vi "displayConfigurableElements.vi"(11 "ConfigurationThisComponent in":refnum<class "ConfigurationThisComponent.lvclass">) -> (3 "ConfigurationThisComponent out":refnum<class "ConfigurationThisComponent.lvclass">)   [LabVIEW 2013, in "ConfigurationThisComponent.lvclass"]
uses:
  ConfigurationThisComponent.lvclass
  <userlib>/Common/ILC/Configuration/ILCSerial.ctl
  <userlib>/Common/SerialProtocols/Configuration/SerialConfig.ctl
  <userlib>/Common/SerialProtocols/Configuration/SerialProtocol.ctl
  <userlib>/Common/SerialProtocols/Configuration/ProtocolParameters.ctl
  <userlib>/Common/SerialProtocols/Configuration/SerialMessageParameters.ctl
  <userlib>/Common/ILC/Configuration/ILCADC.ctl
  <userlib>/Common/ILC/Configuration/InputChannels.ctl
  <userlib>/Common/ILC/Configuration/ScanRate_Hz_MultichannelOptions.ctl
  <userlib>/Common/Devices/FlukeDMM/Config/FlukeDMM.ctl
  <userlib>/Common/SerialProtocols/SerialProtocols.lvlib
  <userlib>/Common/ILC/Configuration/ILCConfiguration.lvlib
  <userlib>/Common/Devices/FlukeDMM/FlukeDMM.lvlib
panel:
  in  "ctrlRefArrayUsrEvnt":refnum<user-event>
  in  "ConfigTab":enum32{"ILC Serial", "ILC ADC", "Fluke DMM"}(tab)
  in  "ILCSerial":T1={"Serial"={"Serial Protocol"=enum."RS485", "Protocol Parameters"={"VISA resource name"="", "Baud Rate"=9600, "Data Bits"=8, "Parity"=enum."None", "Flow Control"=0, "Stop Bits"=10, "Timeout (ms)"=10000}, "Serial Message Parameters"={"Byte Count"=200, "Enable Termination Character"=FALSE, "Termination Char"=200}}} {"Serial"."Serial Message Parameters"."Termination Char" format="%x"; "Serial"."Protocol Parameters"."Stop Bits" items=["1.0"=10, "1.5"=15, "2.0"=20]; "Serial"."Protocol Parameters"."Flow Control" items=["None", "XON/XOFF", "RTS/CTS", "XON/XOFF & RTS/CTS", "DTR/DSR", "XON/XOFF & DTR/DSR"]; "Serial"."Protocol Parameters"."Data Bits" min=5 max=8 step=1}
  in  "ILCADC":T6={"Input Channels"=enum."Channel 0", "Scan Rate (Hz) "=enum."50", "PGA Gain Coefficient"=0, "Reference Voltage Vref"=0.0, "Nominal Input Range in Counts"=128, "Preamplifier Gain"=0, "Conversion Settling Cycles"=0} {"Conversion Settling Cycles" min=1; "Preamplifier Gain" min=1; "Nominal Input Range in Counts" min=128; "Reference Voltage Vref" min=-10.0 max=10.0 format="%.3f"; "PGA Gain Coefficient" max=7}
  in  "FlukeDMM":T9={"Serial"={"Serial Protocol"=enum."RS485", "Protocol Parameters"={"VISA resource name"="", "Baud Rate"=9600, "Data Bits"=8, "Parity"=enum."None", "Flow Control"=0, "Stop Bits"=10, "Timeout (ms)"=10000}, "Serial Message Parameters"={"Byte Count"=200, "Enable Termination Character"=FALSE, "Termination Char"=200}}} {"Serial"."Serial Message Parameters"."Termination Char" format="%x"; "Serial"."Protocol Parameters"."Stop Bits" items=["1.0"=10, "1.5"=15, "2.0"=20]; "Serial"."Protocol Parameters"."Flow Control" items=["None", "XON/XOFF", "RTS/CTS", "XON/XOFF & RTS/CTS", "DTR/DSR", "XON/XOFF & DTR/DSR"]; "Serial"."Protocol Parameters"."Data Bits" min=5 max=8 step=1}
  # "Gain is 2^gain_coefficient"
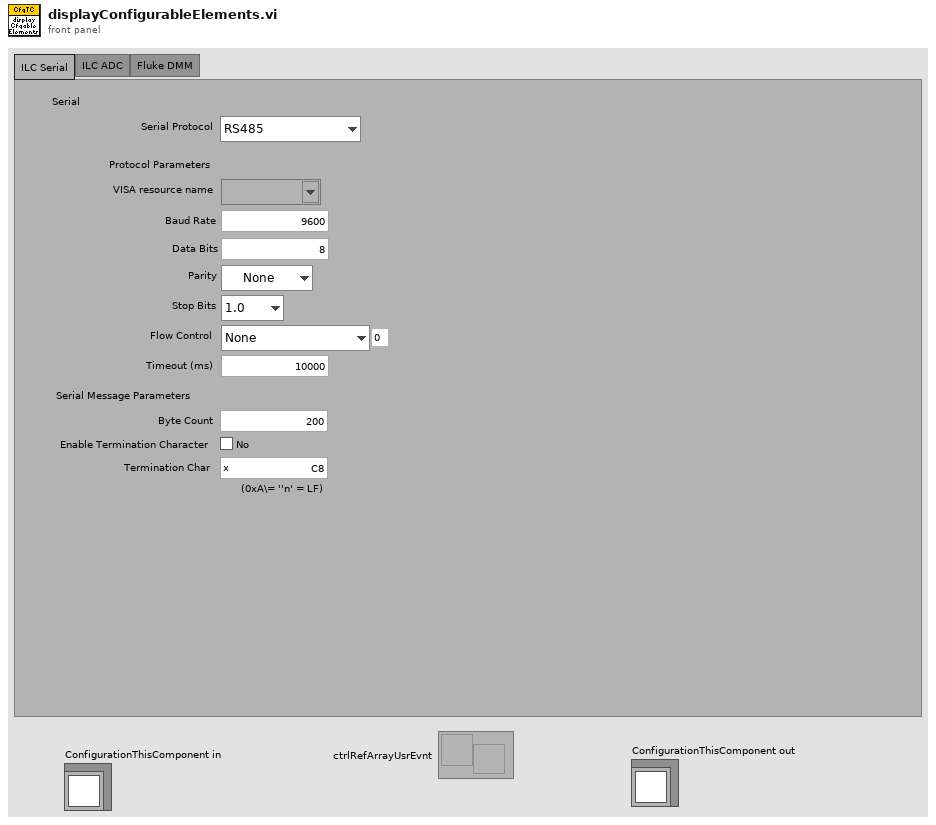
[diagram p1: front panel]
types:
  T1 = typedef "ILCCommon.lvlib/ILCConfiguration.lvlib/ILCSerial.ctl" = cluster{"Serial":T2}
  T2 = typedef "SerialProtocols.lvlib/SerialConfig.ctl" = cluster{"Serial Protocol":T3, "Protocol Parameters":T4, "Serial Message Parameters":T5}
  T3 = typedef "SerialProtocols.lvlib/SerialProtocol.ctl" = enum16{"RS232", "RS485", "SerialSimulator"}
  T4 = typedef "SerialProtocols.lvlib/ProtocolParameters.ctl" = cluster{"VISA resource name":refnum<visa-resource-name>, "Baud Rate":u32, "Data Bits":u16, "Parity":enum16{"None", "Odd", "Even", "Mark", "Space"}, "Flow Control":u16, "Stop Bits":u16, "Timeout (ms)":u32}
  T5 = typedef "SerialProtocols.lvlib/SerialMessageParameters.ctl" = cluster{"Byte Count":u32, "Enable Termination Character":bool, "Termination Char":u8}
  T6 = typedef "ILCCommon.lvlib/ILCConfiguration.lvlib/ILCADC.ctl" = cluster{"Input Channels":T7, "Scan Rate (Hz) ":T8, "PGA Gain Coefficient":u8, "Reference Voltage Vref":dbl[unit], "Nominal Input Range in Counts":u32, "Preamplifier Gain":u8, "Conversion Settling Cycles":u16}
  T7 = typedef "ILCCommon.lvlib/ILCConfiguration.lvlib/InputChannels.ctl" = enum16{"Channel 0", "3 Channels", "5 Channels"}
  T8 = typedef "ILCCommon.lvlib/ILCConfiguration.lvlib/ScanRate_Hz_MultichannelOptions.ctl" = enum16{"50", "60", "100", "120", "200", "240", "300", "400", "480", "600", "1200", "2400", "4800"}
  T9 = typedef "FlukeDMM.lvlib/FlukeDMM.ctl" = cluster{"Serial":T2}
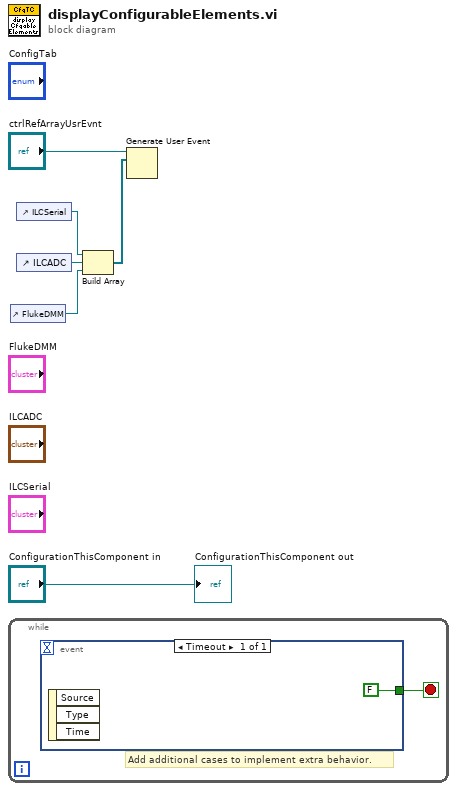
[diagram p0: block diagram]
diagram:
  n1 = while {
    stop <- w7 stop-if-true
    # "Add additional cases to implement extra behavior."
    n2 = event shown="[0] Timeout" {
      selector: _ -> [_]
      dyn-events: _ -> [_]
      timeout: _ -> [_]
      tunnel: [FALSE] -> w7
      event Timeout {
        n3 = event-data() -> ()  [unwired: 1 in, 3 out]
      }
    }
  }
  n4 = control-ref of="FlukeDMM"() -> (w1:refnum<vi>)
  n5 = control-ref of="ILCSerial"() -> (w3:refnum<vi>)
  n6 = control-ref of="ILCADC"() -> (w2:refnum<vi>)
  n7 = Build Array(w3, w2, w1) -> (w6:refnum<vi>[])
  n8 = Generate User Event(user event="ctrlRefArrayUsrEvnt", event data cluster=w6) -> ()  [unwired: 2 in, 2 out]
  "ConfigurationThisComponent out" <- "ConfigurationThisComponent in"
